vi "PathPlanner_Path_PointZoneForWaypointPos.vi"(10 "PointTowardsZone":T1[](array[typedef]) {"TargetPosition"."Y" format="%14.3f"; "TargetPosition"."X" format="%14.3f"; "RotationOffset"."SIN" format="%13.4f"; "RotationOffset"."COS" format="%13.4f"; "RotationOffset"."VALUE" format="%13.4f"}, 11 "Pos":dbl) -> (1 "Found":bool, 3 "outPointTowardsZone":T1={"RotationOffset"={"VALUE"=0.0, "COS"=1.0, "SIN"=0.0}, "Name"="", "TargetPosition"={"X"=0.0, "Y"=0.0}, "MinPosition"=0.0, "MaxPosition"=0.0} {"TargetPosition"."Y" format="%14.3f"; "TargetPosition"."X" format="%14.3f"; "RotationOffset"."SIN" format="%13.4f"; "RotationOffset"."COS" format="%13.4f"; "RotationOffset"."VALUE" format="%13.4f"})   [LabVIEW 2019, in "PathPlanner24.lvlib"]
doc: "This is an internal function. It should not be called by the user.\n\nInputs: \n - pos -\n - PointTowardsZones -\n\nOutputs:\n - outPointTowardsZone\n - found - boolean - TRUE if found."
uses:
  PathPlanner24.lvlib
  TypeDef/PathPlannerPointTowardsZone.ctl
  <vilib>/Rock Robotics/WPI/ThirdParty/JAS_Junk/TrajLib/TypeDef/ROTATION2D.ctl
  <vilib>/Rock Robotics/WPI/ThirdParty/JAS_Junk/TrajLib/TypeDef/TRANSLATION2D.ctl
  <vilib>/Rock Robotics/WPI/ThirdParty/JAS_Junk/TrajLib/Trajectory_Library.lvlib
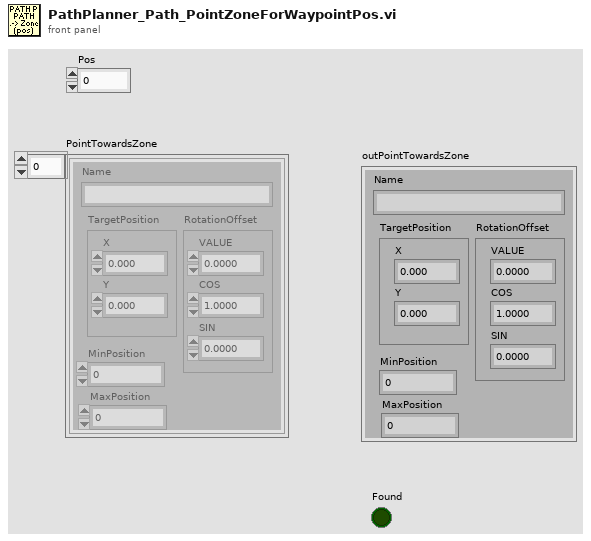
[diagram p1: front panel]
types:
  T1 = typedef "PathPlanner24.lvlib/PathPlannerPointTowardsZone.ctl" = cluster{"RotationOffset":T2, "Name":string, "TargetPosition":T3, "MinPosition":dbl, "MaxPosition":dbl}
  T2 = typedef "Trajectory_Library.lvlib/ROTATION2D.ctl" = cluster{"VALUE":dbl, "COS":dbl, "SIN":dbl}
  T3 = typedef "Trajectory_Library.lvlib/TRANSLATION2D.ctl" = cluster{"X":dbl, "Y":dbl}
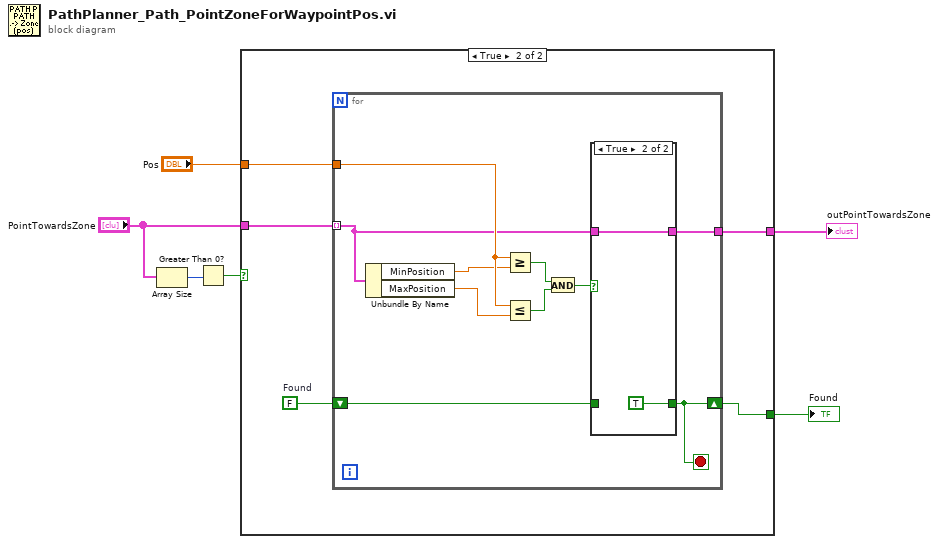
[diagram p0: block diagram]
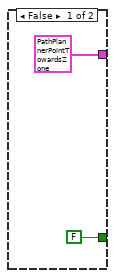
[diagram p2: hidden frame]
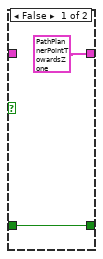
[diagram p3: hidden frame]
diagram:
  n1 = Array Size(array="PointTowardsZone") -> (size(s)=w6:i32)
  n2 = Greater Than 0?(x=w6) -> (x > 0?=w5:bool)
  n3 = case shown="True" w5 {
    tunnel: [T1 {"RotationOffset"={"VALUE"=0.0, "COS"=1.0, "SIN"=0.0}, "Name"="", "TargetPosition"={"X"=0.0, "Y"=0.0}, "MinPosition"=0.0, "MaxPosition"=0.0} ("outPointTowardsZone") w9] -> w4
    tunnel: [FALSE ("Found") w11] -> w3
    tunnel: "PointTowardsZone" -> [_ w13]
    tunnel: "Pos" -> [_ w10]
    frame False {
    }
    frame True {
      w12 = FALSE  # Found
      n4 = for {
        tunnel: w13 -> [w14] mode=indexing
        shift-right: [w17] -> w11
        shift-left: w12 -> [w16]
        tunnel: w10 -> [w23]
        tunnel: [w15] -> w9
        stop <- w17 stop-if-true
        n5 = Unbundle By Name(w14) -> ("MinPosition"=w22:dbl, "MaxPosition"=w21:dbl)
        n6 = Greater Or Equal?(x=w23, y=w22) -> (x >= y?=w20:bool)
        n7 = Less Or Equal?(x=w23, y=w21) -> (x <= y?=w19:bool)
        n8 = And(x=w20, y=w19) -> (x .and. y?=w18:bool)
        n9 = case shown="True" w18 {
          tunnel: [w25 TRUE] -> w17
          tunnel: w16 -> [w25 _]
          tunnel: [T1 {"RotationOffset"={"VALUE"=0.0, "COS"=1.0, "SIN"=0.0}, "Name"="", "TargetPosition"={"X"=0.0, "Y"=0.0}, "MinPosition"=0.0, "MaxPosition"=0.0} ("outPointTowardsZone") w26] -> w15
          tunnel: w14 -> [_ w26]
          frame False {
          }
          frame True {
          }
        }
      }
    }
  }
  "outPointTowardsZone" <- w4
  "Found" <- w3
